vi "主程序-复材超声C扫缺陷分析评定软件.vi"() -> ()   [LabVIEW 2018]
doc: "使用该模板构建用户界面事件处理设计模式。将模板应用于对话框及其它用户界面。用户也可创建并执行VI可按照与用户界面事件相同方式处理的用户定义事件。"
uses:
  <vilib>/Utility/NIReport.llb/Report Type.ctl
  <vilib>/addons/_office/_exclsub.llb/font.ctl
  <vilib>/Utility/NIReport.llb/HTML Report Image Alignment.ctl
  <vilib>/Utility/NIReport.llb/Append Report Text (str wrap).vi
  <vilib>/Utility/NIReport.llb/Append Image to Report (path wrap).vi
  <vilib>/addons/_office/word.llb/Word Easy Table (str).vi
  <vilib>/Utility/NIReport.llb/NI_report.lvclass
  <vilib>/Utility/NIReport.llb/Word/NI_Word.lvclass
  <vilib>/addons/_office/NI_ReportGenerationToolkit.lvlib
  <vilib>/Utility/NIReport.llb/NI_ReportGenerationCore.lvlib
  <vilib>/vision/NI_Vision_Development_Module.lvlib
panel:
  out "flag数组":i8[](array[numeric])
  out "字符串":string
  out "图像Y向分辨率（mm/像素）":dbl
  out "图像X向分辨率（mm/像素）":dbl
  out "判定为筋条的长宽比阈值":i32
  out "框号字体大小-":i16
  out "是否需要预处理":u16
  out "计入缺陷的Z值阈值":i32 caption="值"
  out "计入缺陷的面积阈值":i32
  out "报告模式":string
  in  "删除标注":bool caption="定量分析"
  out "缺陷灰度阈值":dbl caption="值"
  out "穿透图原始路径":path
  out "ROImask":T1(plugin-control)
  out "添加的路径":path
  out "连接的字符串 2":string
  out "临界面积百分比值":dbl
  out "临界Z值":i32
  out "标注后的图片路径":path
  out "全部检测结果合并":string[][](table)
  out "全部检测结果":string[][](table)
  out "部位信息":string[](array[string])=["", "34.500000", "32.500000", "1121", "34", "54.955926", "分层类", "不合格", ""]
  in  "完成标注":bool caption="定量分析"
  out "框数":dbl
  out "自定义字体":T2={"Desired Font (Application)"=enum."Application Font", "[User-specified Font]"={"Font Name"="", "Size"=12, "Strikeout?"=FALSE, "Italic?"=FALSE, "Underline?"=FALSE, "Outline?"=FALSE, "Shadow?"=FALSE, "Bold?"=FALSE, "Rotation Angle"=0.0}, "Horizontal Alignment"=0, "Vertical Alignment"=0} {"Horizontal Alignment" items=["Left", "Center", "Right"]; "Vertical Alignment" items=["Bottom", "Top", "Baseline"]}
  out "框组":T3(array[cluster])
  out "质量等级":string
  in  "stop":bool caption="停止"
  in  "导入图像":bool caption="导入图片"
  in  "开始标注":bool caption="定量分析"
  in  "查看评定结果":bool caption="辅助定性分析"
  in  "生成报告":bool caption="生成原始记录"
  in  "控件":enum32{"穿透图"}(tab)
  out "穿透图":T1(plugin-control)
  out "产品规格":cluster{"产品长度（周长）（mm）":dbl, "产品宽度（母线长）（mm）":dbl}
  out "图像分辨率":T4
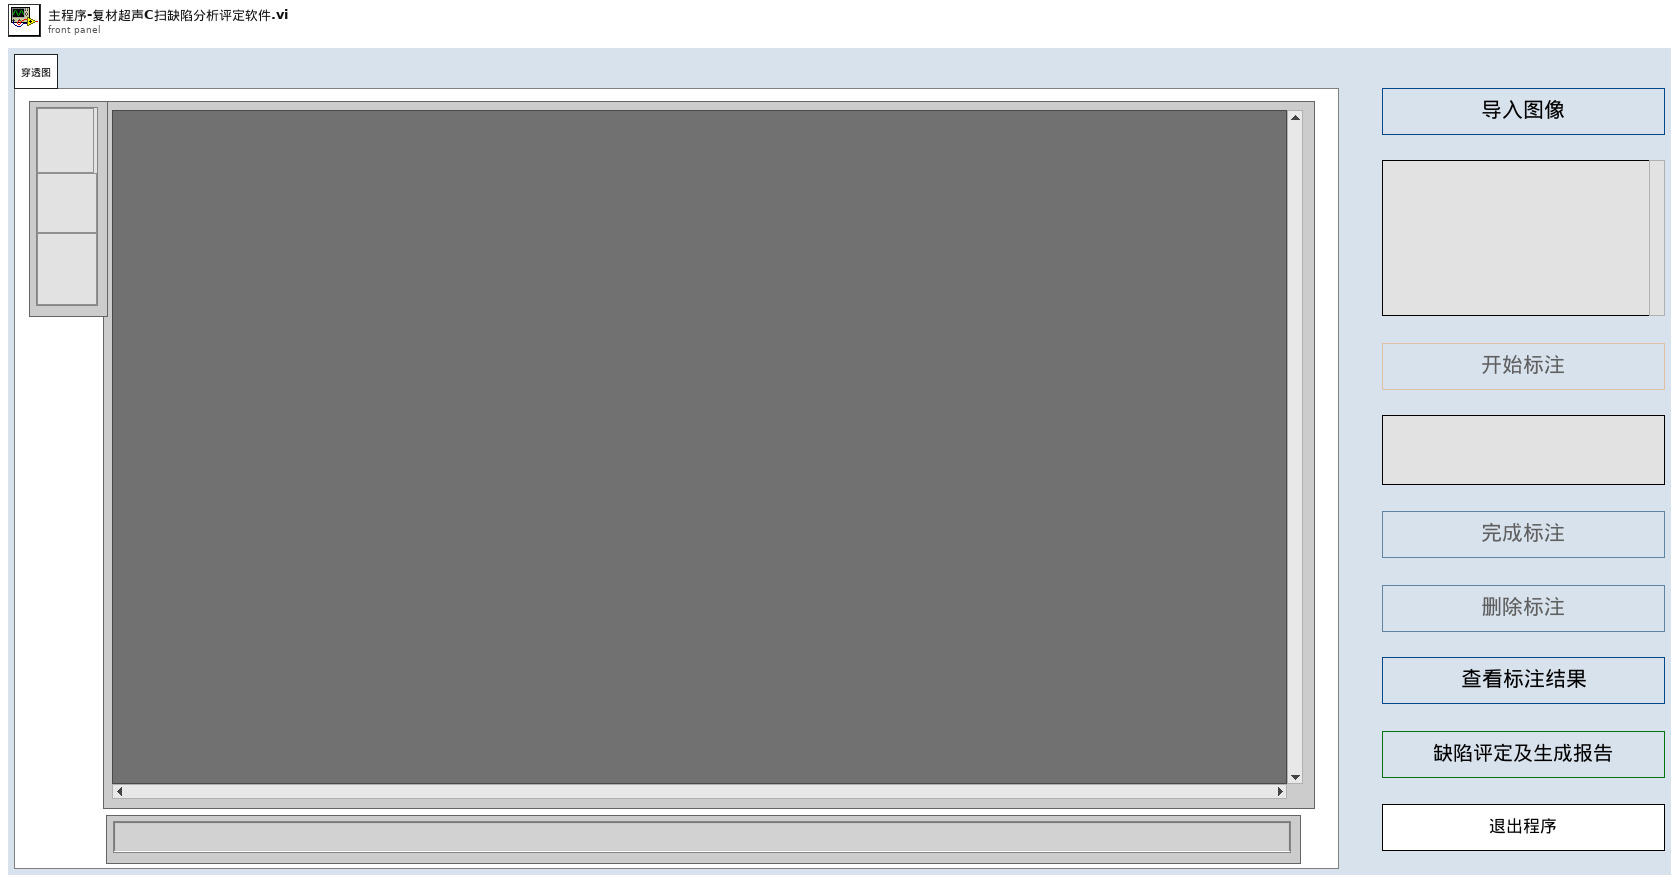
[diagram p1: front panel]
types:
  T1 = typedef "IMAQ Image.ctl" = refnum<image>
  T2 = cluster{"Desired Font (Application)":enum16{"User-specified Font", "Application Font", "System Font", "Dialog Font"}, "[User-specified Font]":cluster{"Font Name":string, "Size":i16, "Strikeout?":bool, "Italic?":bool, "Underline?":bool, "Outline?":bool, "Shadow?":bool, "Bold?":bool, "Rotation Angle":dbl}, "Horizontal Alignment":i16, "Vertical Alignment":i16}
  T3 = cluster{"Global Rectangle":i32[], "Contours":cluster{"Contour Type":u32, "ROI Type":u32, "Points":i32[]}[]}[]
  T4 = cluster{"图像X向分辨率（mm/像素）":dbl, "图像Y向分辨率（mm/像素）":dbl}
  T5 = enum8{"Enabled", "Disabled", "Disabled and Grayed Out"}
  T6 = cluster{"Global Rectangle":i32[], "Contours":cluster{"Contour Type":u32, "ROI Type":u32, "Points":i32[]}[]}
  T7 = cluster{"Zoom Tool":bool, "Selection Tool":bool, "Pan Tool":bool, "Point Tool":bool, "Line Tool":bool, "Rectangle Tool":bool, "Rotated Rectangle Tool":bool, "Polyline Tool":bool, "Polygon Tool":bool, "Freehand Tool":bool, "Closed Freehand Tool":bool, "Ellipse Tool":bool, "Annulus Tool":bool}
  T8 = enum16{"maximized", "minimized", "normal", "no change"}
  T9 = typedef "NI_ReportGenerationCore.lvlib/Report Type.ctl" = enum16{"HTML", "Word", "Excel"}
  T10 = typedef "NI_ReportGenerationCore.lvlib/HTML Report Image Alignment.ctl" = enum16{"(default)", "LEFT", "RIGHT", "TOP", "TEXTTOP", "MIDDLE", "ABSMIDDLE", "BASELINE", "BOTTOM", "ABSBOTTOM"}
  T11 = cluster{"position (Excel)":cluster{"row":i32, "column":i32}, "name (Excel)":string, "bookmark (Word)":string}
  T12 = cluster{"position (excel)":cluster{"row":i32, "column":i32}, "name (excel)":string, "bookmark (word)":string}
  T13 = typedef "NI_ReportGenerationToolkit.lvlib/font.ctl" = cluster{"font name":string, "font size":dbl, "bold":u16, "italic":u16, "underline":u16, "strike through":u16, "font color":u32}
  T14 = typedef "Image Type" = u32
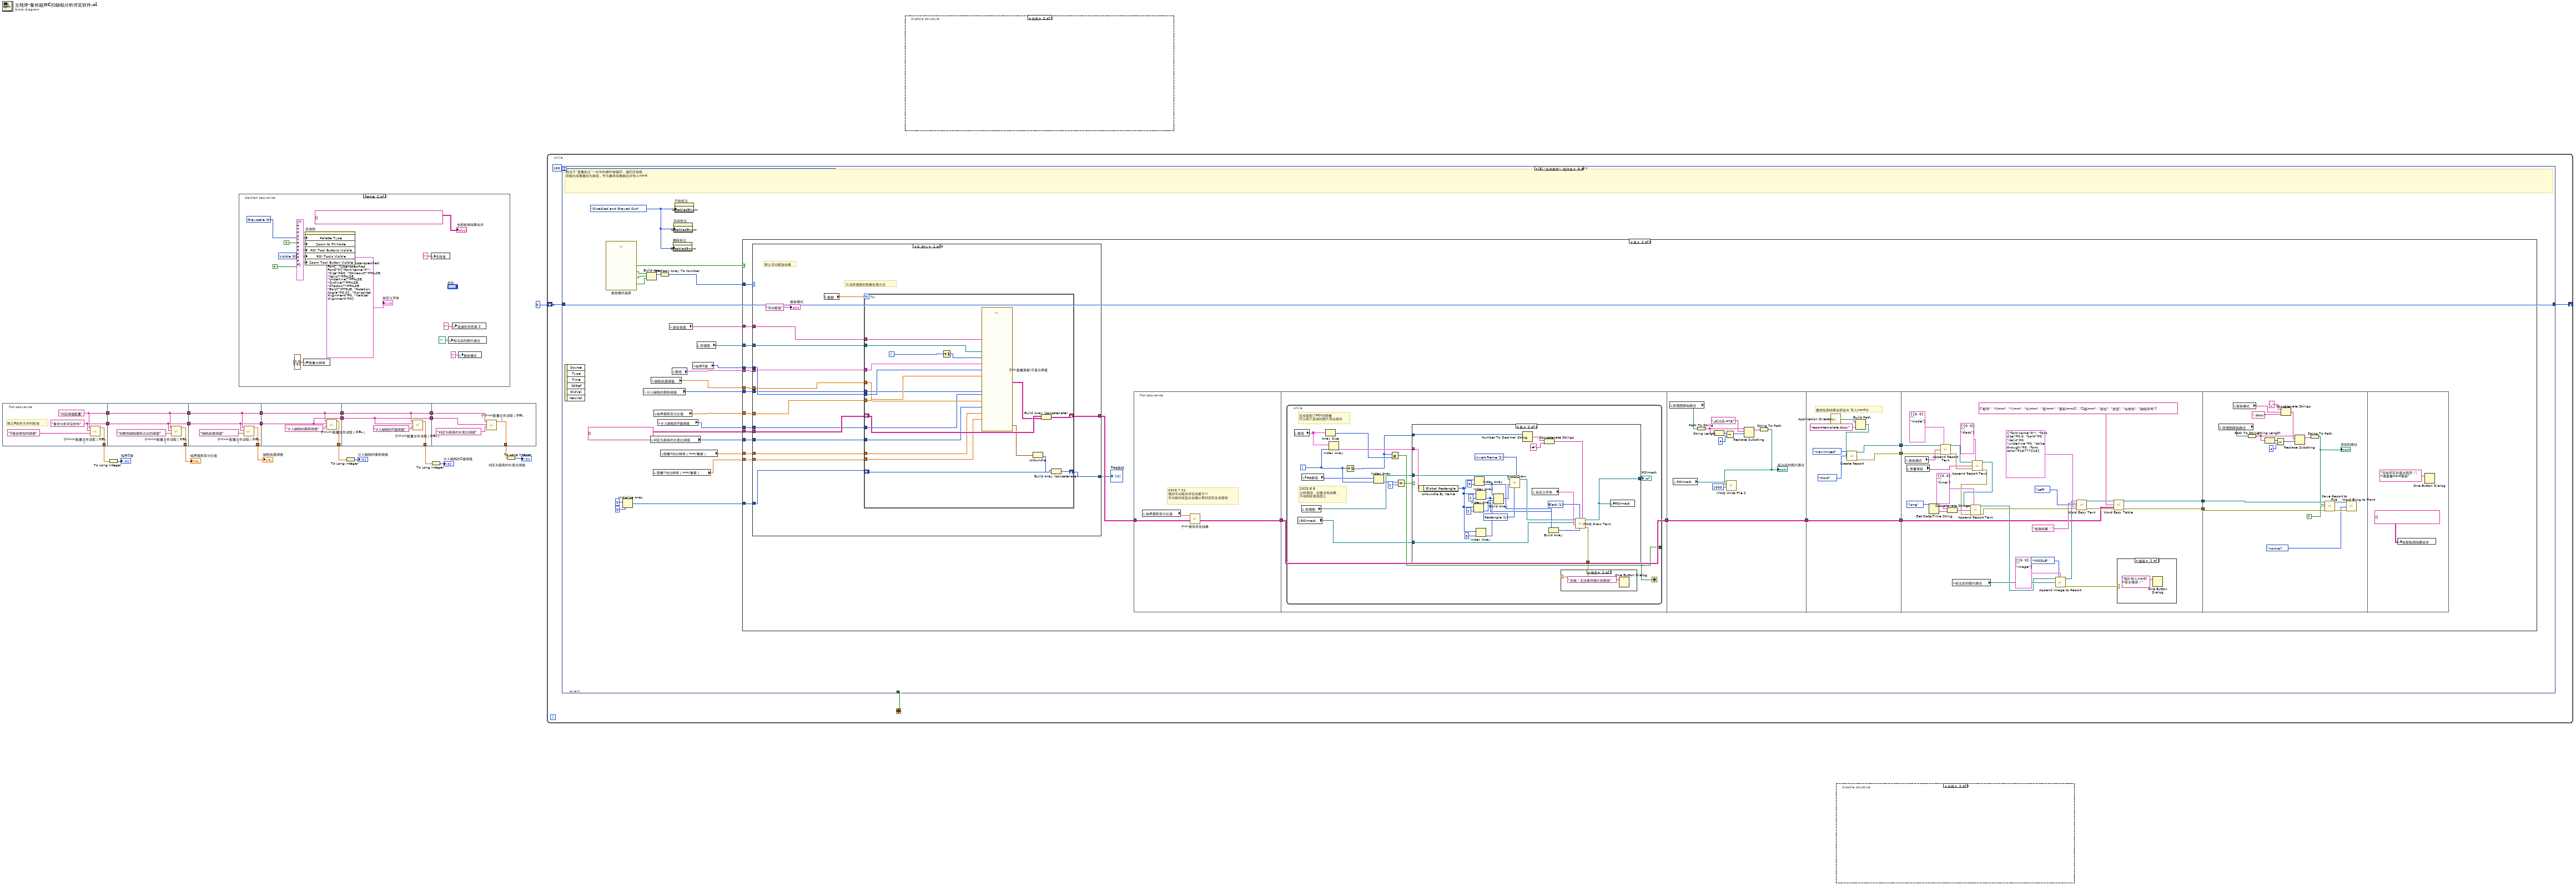
[diagram p0: block diagram]
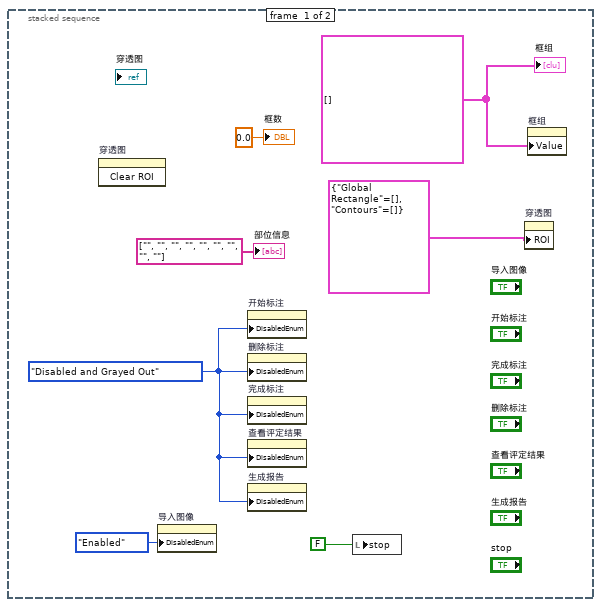
[diagram p3: hidden frame]
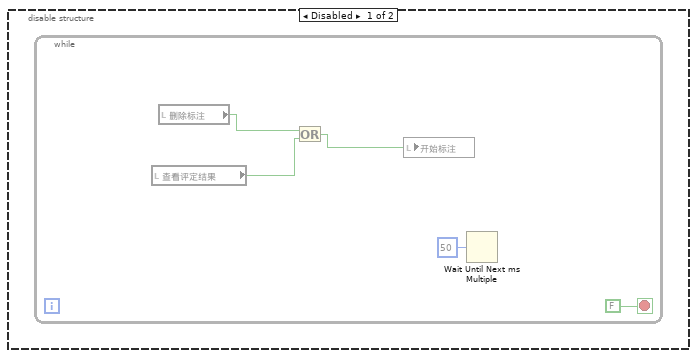
[diagram p4: hidden frame]
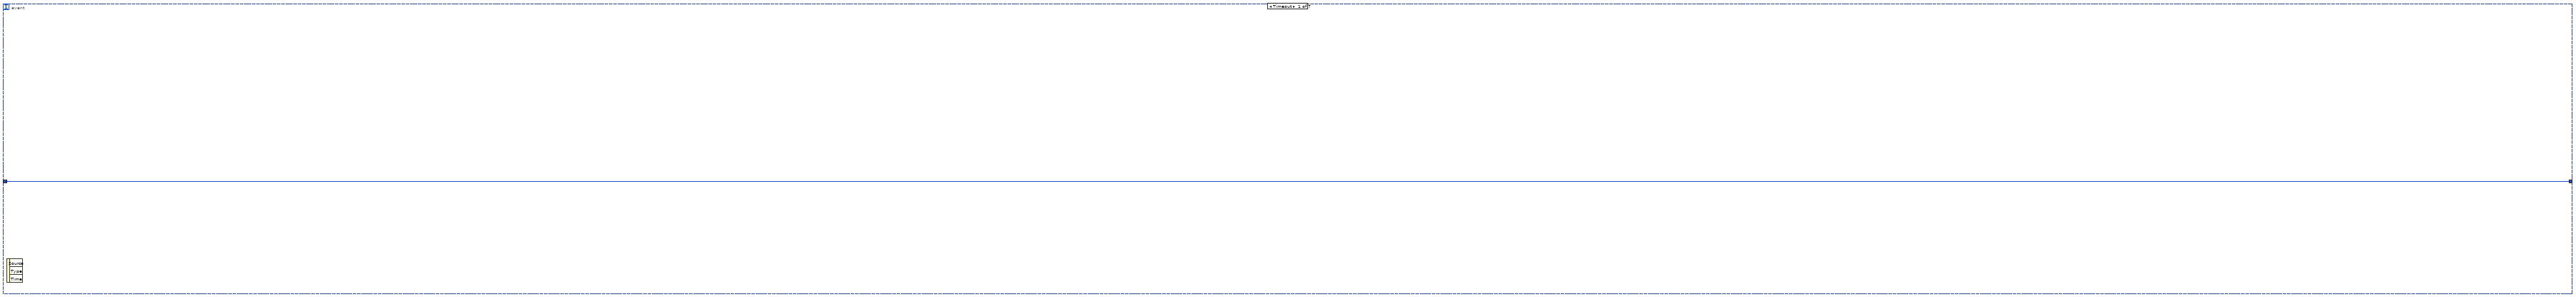
[diagram p5: hidden frame]
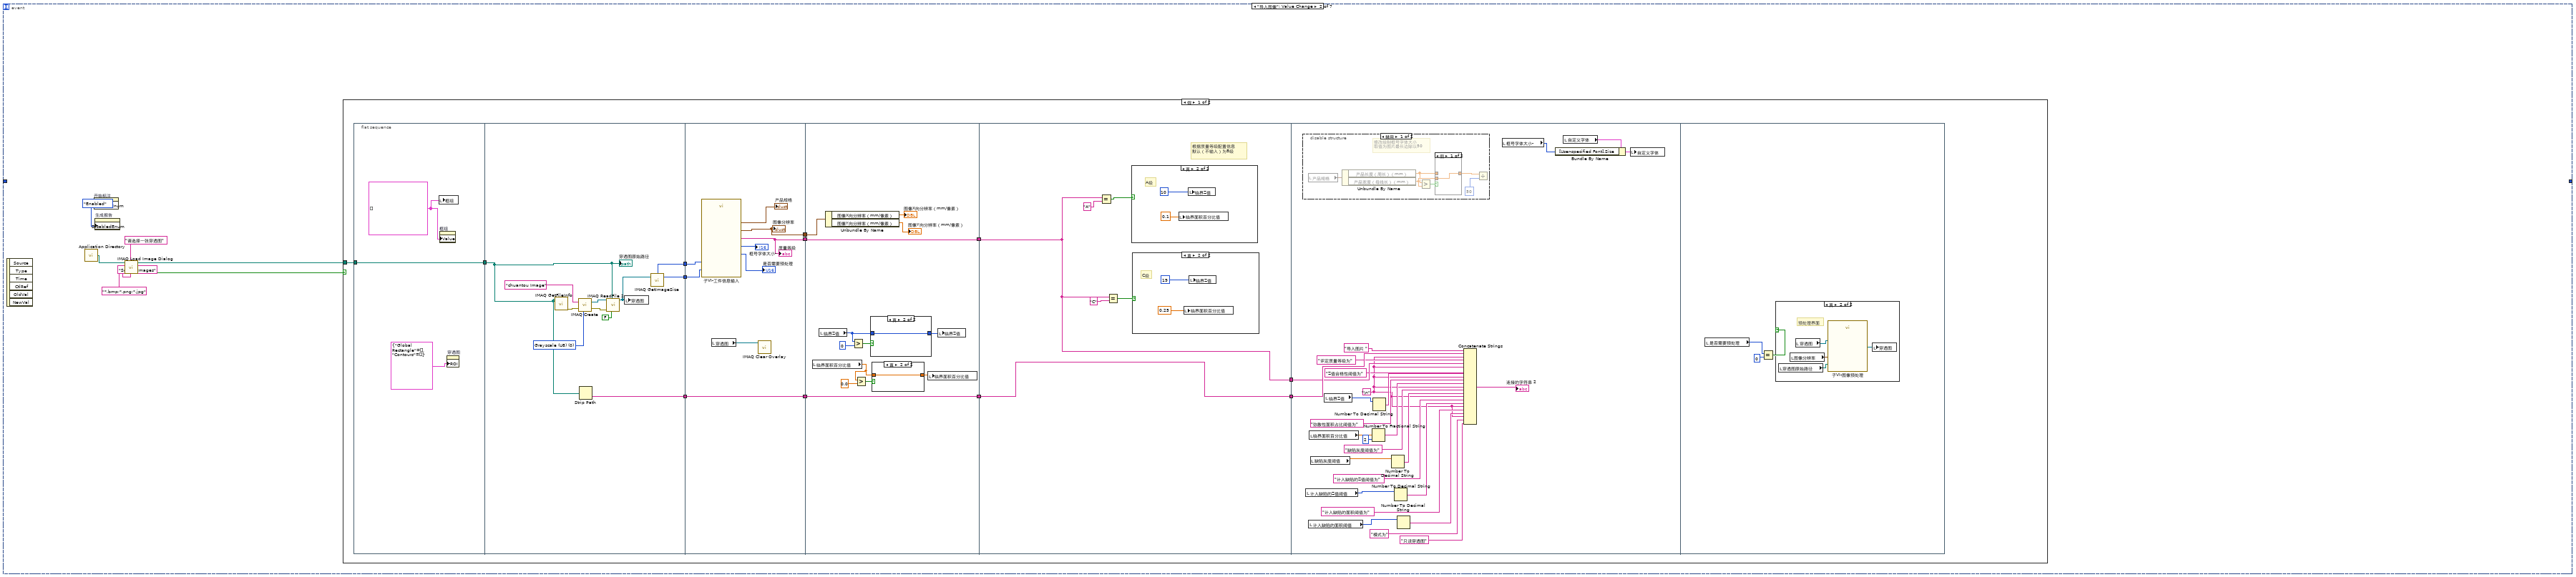
[diagram p6: hidden frame]
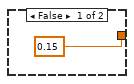
[diagram p7: hidden frame]
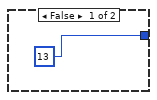
[diagram p8: hidden frame]
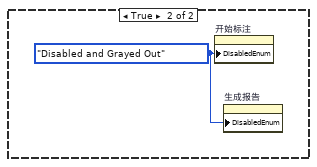
[diagram p14: hidden frame]
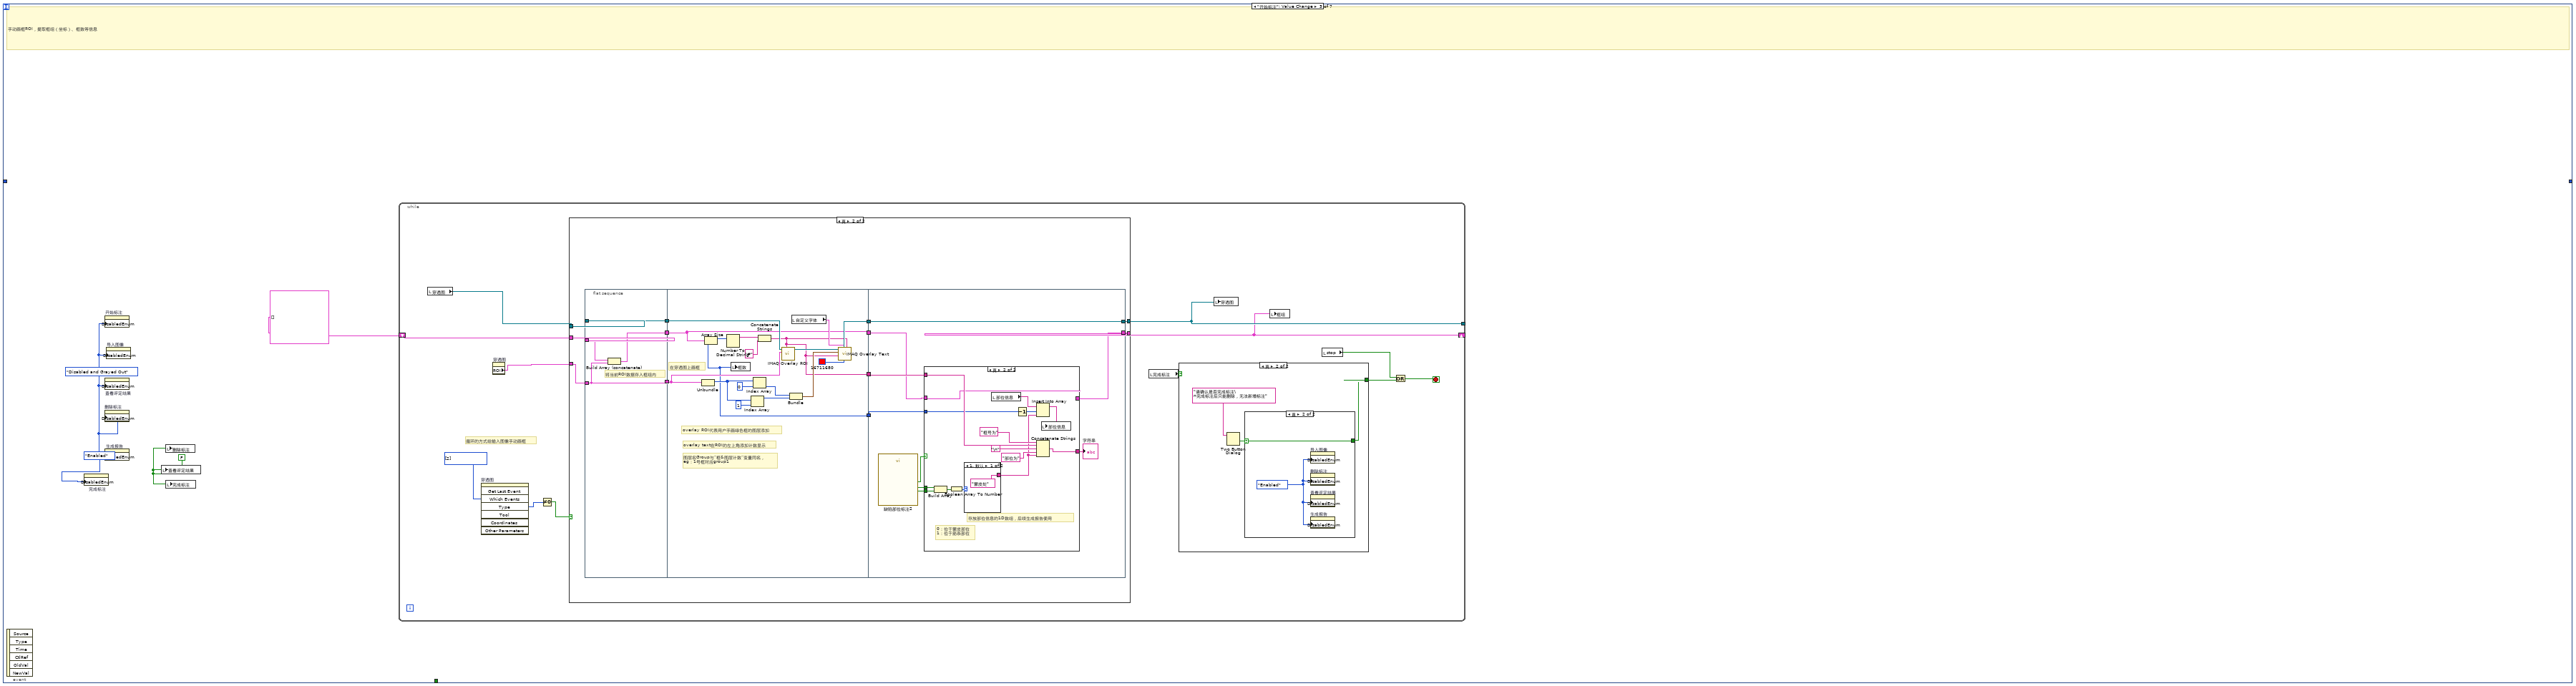
[diagram p15: hidden frame]
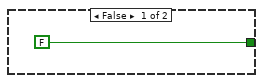
[diagram p16: hidden frame]
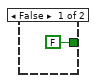
[diagram p17: hidden frame]
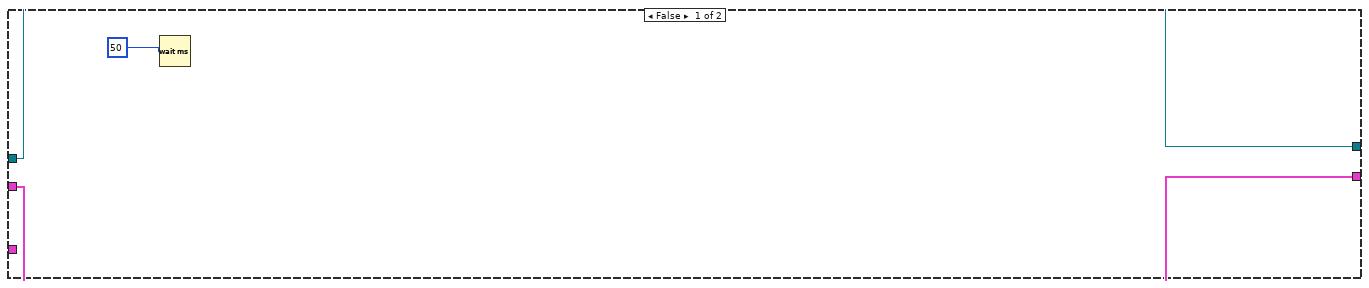
[diagram p18: hidden frame]
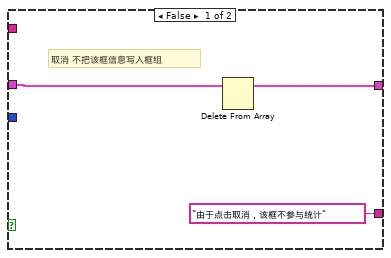
[diagram p19: hidden frame]
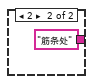
[diagram p20: hidden frame]
diagram:
  n1 = flat-sequence {
    tunnel: [w24] -> w20
    tunnel: [w23] -> w19
    tunnel: [w22] -> w14
    tunnel: w20 -> [w27]
    tunnel: w19 -> [w28]
    tunnel: [w28] -> w18
    tunnel: [w27] -> w17
    tunnel: [w26] -> w15
    tunnel: w18 -> [w30]
    tunnel: w17 -> [w31]
    tunnel: [w32] -> w16
    tunnel: [w31] -> w12
    tunnel: [w30] -> w11
    tunnel: w12 -> [w35]
    tunnel: w11 -> [w34]
    tunnel: [w36] -> w9
    tunnel: [w35] -> w8
    tunnel: [w34] -> w7
    tunnel: w8 -> [w39]
    tunnel: w7 -> [w38]
    tunnel: [w40] -> w5
    tunnel: [w39] -> w4
    tunnel: [w38] -> w3
    tunnel: w4 -> [w45]
    tunnel: w3 -> [w44]
    tunnel: [w42] -> w2
    frame #0 {
      w23 = "复材分析评定软件" ("section")
      w24 = "判定阈值配置" ("文件名称")
      # "默认B级作为评判标准"
      n2 = call "子VI-ini配置文件读取（DBL）.vi"("key"="Z值合格性的阈值", "section"=w23, "文件名称"=w24) -> ("value"=w22:dbl)  [unwired: 8 in]
    }
    frame #1 {
      n3 = call "子VI-ini配置文件读取（DBL）.vi"("key"="弥散性缺陷面积占比的阈值", "section"=w28, "文件名称"=w27) -> ("value"=w26:dbl)  [unwired: 8 in]
    }
    frame #2 {
      n4 = call "子VI-ini配置文件读取（DBL）.vi"("key"="缺陷灰度阈值", "section"=w30, "文件名称"=w31) -> ("value"=w32:dbl)  [unwired: 8 in]
    }
    frame #3 {
      n5 = call "子VI-ini配置文件读取（DBL）.vi"("key"="计入缺陷的面积阈值", "section"=w34, "文件名称"=w35) -> ("value"=w36:dbl)  [unwired: 8 in]
    }
    frame #4 {
      n6 = call "子VI-ini配置文件读取（DBL）.vi"("key"="计入缺陷的Z值阈值", "section"=w38, "文件名称"=w39) -> ("value"=w40:dbl)  [unwired: 8 in]
    }
    frame #5 {
      n7 = call "子VI-ini配置文件读取（DBL）.vi"("key"="判定为筋条的长宽比阈值", "section"=w44, "文件名称"=w45) -> ("value"=w42:dbl)  [unwired: 8 in]
    }
  }
  n8 = To Long Integer(number=w14) -> (32bit integer=→"临界Z值":i32)
  n9 = stacked-sequence {
    frame #0 {
      w50 = T3 [] ("框组")
      w48 = T5."Disabled and Grayed Out" ("禁用")
      n10 = invoke on="穿透图" class="ImageControl" method="Clear ROI"() -> ()  [unwired: 3 in, 3 out]
      n11 = property on="导入图像" class="Bool"("DisabledEnum"=T5."Enabled" ("禁用")) -> ()  [unwired: 2 in, 2 out]
      n12 = property on="开始标注" class="Bool"("DisabledEnum"=w48) -> ()  [unwired: 2 in, 2 out]
      n13 = property on="删除标注" class="Bool (严格)"("DisabledEnum"=w48) -> ()  [unwired: 2 in, 2 out]
      n14 = property on="完成标注" class="Bool (严格)"("DisabledEnum"=w48) -> ()  [unwired: 2 in, 2 out]
      n15 = property on="查看评定结果" class="Bool (严格)"("DisabledEnum"=w48) -> ()  [unwired: 2 in, 2 out]
      n16 = property on="生成报告" class="Bool"("DisabledEnum"=w48) -> ()  [unwired: 2 in, 2 out]
      n17 = local write "stop"(FALSE ("stop")) -> ()
      n18 = property on="穿透图" class="ImageControl"("ROI"=T6 {"Global Rectangle"=[], "Contours"=[]}) -> ()  [unwired: 2 in, 2 out]
      n19 = property on="框组" class="Arr (严格)"("Value"=w50) -> ()  [unwired: 2 in, 2 out]
      "部位信息" <- string[] ["", "", "", "", "", "", "", "", ""] ("部位信息")
      "框组" <- w50
      "框数" <- 0.0 ("框数")
    }
    frame #1 {
      w54 = u32 0 items=["Visible", "Hidden", "Hidden, Use WindTools Palette"] ("ROI Tools Visible")
      w57 = u32 0 items=["Grayscale", "Binary", "Gradient", "Rainbow", "Temperature", "User Defined", "Binary 16 Bit", "Gradient 16 Bit", "Rainbow 16 Bit", "Temperature 16 Bit", "User Defined 16 Bit"] ("Palette:Palette Type")
      n20 = local write "图像分辨率"(T4 {"图像X向分辨率（mm/像素）"=1.0, "图像Y向分辨率（mm/像素）"=1.0} ("图像分辨率")) -> ()
      n21 = property on="穿透图" class="ImageControl"("Palette Type"=w57, "Zoom to Fit Mode"=TRUE, "ROI Tool Buttons Visible"=T7 {"Zoom Tool"=TRUE, "Selection Tool"=FALSE, "Pan Tool"=TRUE, "Point Tool"=FALSE, "Line Tool"=FALSE, "Rectangle Tool"=TRUE, "Rotated Rectangle Tool"=FALSE, "Polyline Tool"=FALSE, "Polygon Tool"=FALSE, "Freehand Tool"=FALSE, "Closed Freehand Tool"=FALSE, "Ellipse Tool"=FALSE, "Annulus Tool"=FALSE} ("ROI Tool Buttons Visible:All Elements"), "ROI Tools Visible"=w54, "Zoom Tool Button Visible"=TRUE ("ROI Tool Buttons Visible:Zoom Tool Button Visible")) -> ()  [unwired: 2 in, 2 out]
      n22 = local write "字符串"("" ("字符串")) -> ()
      n23 = local write "标注后的图片路径"(path "" ("标注后的图片路径")) -> ()
      n24 = local write "连接的字符串 2"("" ("连接的字符串 2")) -> ()
      n25 = local write "报告模式"("" ("报告模式")) -> ()
      "自定义字体" <- T2 {"Desired Font (Application)"=enum."User-specified Font", "[User-specified Font]"={"Font Name"="", "Size"=60, "Strikeout?"=FALSE, "Italic?"=FALSE, "Underline?"=FALSE, "Outline?"=FALSE, "Shadow?"=FALSE, "Bold?"=TRUE, "Rotation Angle"=0.0}, "Horizontal Alignment"=0, "Vertical Alignment"=0} ("Font, Size & Style")
      "全部检测结果合并" <- string[][] [] ("弥散类检测结果合并")
    }
  }
  n26 = To Long Integer(number=w9) -> (32bit integer=→"计入缺陷的面积阈值":i32)
  n27 = To Long Integer(number=w5) -> (32bit integer=→"计入缺陷的Z值阈值":i32)
  n28 = To Long Integer(number=w2) -> (32bit integer=→"判定为筋条的长宽比阈值":i32)
  n29 = while {
    shift-right: [w65] -> _
    shift-left: 0 -> [w66]
    stop <- w68 stop-if-true
    n30 = event shown="[5] \"生成报告\": 值改变" {
      selector: _ -> [_ _ _ _ _ _ _]
      dyn-events: _ -> [_ _ _ _ _ _ _]
      timeout: 100 -> [_ _ _ _ _ _ _]
      tunnel: [_ _ _ _ _ _ w585] -> w68
      tunnel: w66 -> [w69 _ _ _ _ w339 _]
      tunnel: [w69 _ _ _ _ w339 0] -> w65
      event Timeout {
        n31 = event-data() -> ()  [unwired: 1 in, 3 out]
      }
      event "导入图像": Value Change {
        w71 = T5."Enabled" ("禁用")
        n32 = event-data() -> ()  [unwired: 1 in, 6 out]
        n33 = call <vilib>:"Application Directory.vi"() -> ("Application Directory"=w70:path)
        n34 = property on="开始标注" class="Bool"("DisabledEnum"=w71) -> ()  [unwired: 2 in, 2 out]
        n35 = property on="生成报告" class="Bool"("DisabledEnum"=w71) -> ()  [unwired: 2 in, 2 out]
        n36 = call "IMAQ Load Image Dialog"("Pattern Label"="Source Images", "Prompt"="请选择一张穿透图" ("prompt"), "Pattern"="*.bmp;*.png;*.jpg", "Start Path"=w70) -> ("Cancelled?"=w73:bool, "Path"=w72:path)  [unwired: 5 in, 1 out]
        n37 = case shown="假" w73 {
          tunnel: w72 -> [w86 _]
          frame False {
            n38 = flat-sequence {
              tunnel: w86 -> [w90]
              tunnel: [w90] -> w85
              tunnel: w85 -> [w93]
              tunnel: [w95] -> w84
              tunnel: [w94] -> w83
              tunnel: [w92] -> w82
              tunnel: [w110] -> w88
              tunnel: w84 -> [w109]
              tunnel: w83 -> [w108]
              tunnel: w82 -> [w107]
              tunnel: [w107] -> w81
              tunnel: [w103] -> w77
              tunnel: w88 -> [w124]
              tunnel: [w124] -> w87
              tunnel: w81 -> [w123]
              tunnel: [w123] -> w80
              tunnel: w77 -> [w114]
              tunnel: w87 -> [w129]
              tunnel: w80 -> [w130]
              tunnel: [w130] -> w79
              tunnel: [w129] -> w78
              tunnel: w79 -> [w156]
              tunnel: w78 -> [w154]
              frame #0 {
                w91 = T3 [] ("框组")
                n39 = local write "框组"(w91) -> ()
                n40 = property on="框组" class="Arr (严格)"("Value"=w91) -> ()  [unwired: 2 in, 2 out]
                n41 = property on="穿透图" class="ImageControl"("ROI"=T6 {"Global Rectangle"=[], "Contours"=[]}) -> ()  [unwired: 2 in, 2 out]
              }
              frame #1 {
                w97 = T14 0 items=["Grayscale (U8)", "Grayscale (I16)", "Grayscale (SGL)", "Complex (CSG)", "RGB (U32)", "HSL (U32)", "RGB (U64)", "Grayscale (U16)"] ("Image Type")
                n42 = call "IMAQ GetFileInfo"("File Path"=w93) -> ("error out"=w100:errorcluster)  [unwired: 4 in, 6 out]
                n43 = call "IMAQ Create"("Image Name"="chuantou Image", "Image Type"=w97, "error in (no error)"=w100) -> ("New Image"=w101:T1, "error out"=w102:errorcluster)  [unwired: 2 in]
                n44 = Strip Path(path=w93) -> (name=w92:string)  [unwired: 1 out]
                n45 = call "IMAQ ReadFile 2"("Use File Path Image Type"=FALSE, "File Path"=w93, "error in (no error)"=w102, "Image"=w101) -> ("Image Out"=w99:T1)  [unwired: 3 in, 4 out]
                n46 = local write "穿透图"(w99) -> ()
                n47 = call "IMAQ GetImageSize"("Image"=w99) -> ("Y Resolution"=w94:i32, "X Resolution"=w95:i32)  [unwired: 3 in, 1 out]
                "穿透图原始路径" <- w93
              }
              frame #2 {
                n48 = call "子VI-工件信息输入.vi"("Y Resolution"=w108, "X Resolution"=w109) -> ("质量等级"=w110:string, "框号字体大小-"=→"框号字体大小-":i16, "产品规格"=→"产品规格":cluster{"产品长度（周长）（mm）":dbl, "产品宽度（母线长）（mm）":dbl}, "是否需要预处理"=→"是否需要预处理":u16, "图像分辨率"=w103:T4)  [unwired: 5 in]
                "图像分辨率" <- w103
                "质量等级" <- w110
                n49 = local read "穿透图"() -> (w106:T1)
                n50 = call "IMAQ Clear Overlay"("Image"=w106) -> ()  [unwired: 9 in, 2 out]
              }
              frame #3 {
                n51 = local read "临界面积百分比值"() -> (w115:dbl)
                n52 = local read "临界Z值"() -> (w116:i32)
                n53 = Unbundle By Name(w114) -> ("图像X向分辨率（mm/像素）"=→"图像X向分辨率（mm/像素）":dbl, "图像Y向分辨率（mm/像素）"=→"图像Y向分辨率（mm/像素）":dbl)
                n54 = Greater?(x=w116, y=0) -> (0:w121:bool)
                n55 = Greater?(x=w115, y=0.0) -> (0:w119:bool)
                n56 = case shown="真" w121 {
                  tunnel: [13 ("临界Z值") w128] -> w118
                  tunnel: w116 -> [_ w128]
                  frame False {
                  }
                  frame True {
                  }
                }
                n57 = case shown="真" w119 {
                  tunnel: [0.15 ("临界面积百分比值") w126] -> w117
                  tunnel: w115 -> [_ w126]
                  frame False {
                  }
                  frame True {
                  }
                }
                n58 = local write "临界面积百分比值"(w117) -> ()
                n59 = local write "临界Z值"(w118) -> ()
              }
              frame #4 {
                # "根据质量等级配置信息\n默认（不输入）为B级"
                n60 = Equal?(x=w129, y="A") -> (x = y?=w133:bool)
                n61 = Equal?(x=w129, y="C") -> (x = y?=w134:bool)
                n62 = case shown="真" w133 {
                  frame False {
                  }
                  frame True {
                    # "A级"
                    n63 = local write "临界面积百分比值"(0.1 ("临界面积百分比值")) -> ()
                    n64 = local write "临界Z值"(10 ("临界Z值")) -> ()
                  }
                }
                n65 = case shown="真" w134 {
                  frame False {
                  }
                  frame True {
                    # "C级"
                    n66 = local write "临界面积百分比值"(0.25 ("临界面积百分比值")) -> ()
                    n67 = local write "临界Z值"(19 ("临界Z值")) -> ()
                  }
                }
              }
              frame #5 {
                w144 = "\n"
                n68 = disable-structure shown="禁用" {
                  frame Disabled {
                    # "修改绘制框号字体大小\n取值为图片最长边除以50"
                    n69 = local read "产品规格"() -> (w167:cluster{"产品长度（周长）（mm）":dbl, "产品宽度（母线长）（mm）":dbl})
                    n70 = Unbundle By Name(w167) -> ("产品长度（周长）（mm）"=w169:dbl, "产品宽度（母线长）（mm）"=w170:dbl)
                    n71 = Greater?(x=w169, y=w170) -> (0:w168:bool)
                    n72 = case shown="假" w168 {
                      tunnel: w169 -> [_ w173]
                      tunnel: w170 -> [w172 _]
                      tunnel: [w172 w173] -> w171
                      frame False {
                      }
                      frame True {
                      }
                    }
                    n73 = Divide(x=w171, y=i8 50) -> ()  [unwired: 1 out]
                  }
                  frame Enabled {
                  }
                }
                n74 = local read "计入缺陷的Z值阈值"() -> (w150:i32)
                n75 = local read "计入缺陷的面积阈值"() -> (w147:i32)
                n76 = local read "临界面积百分比值"() -> (w162:dbl)
                n77 = local read "缺陷灰度阈值"() -> (w164:dbl)
                n78 = local read "临界Z值"() -> (w160:i32)
                n79 = Number To Fractional String(number=w162, precision (6)=i16 2 ("精度(6)")) -> (F-format string=w163:string)  [unwired: 2 in]
                n80 = Number To Decimal String(number=w160) -> (decimal integer string=w161:string)  [unwired: 1 in]
                n81 = Number To Decimal String(number=w164) -> (decimal integer string=w165:string)  [unwired: 1 in]
                n82 = Number To Decimal String(number=w150) -> (decimal integer string=w148:string)  [unwired: 1 in]
                n83 = Number To Decimal String(number=w147) -> (decimal integer string=w145:string)  [unwired: 1 in]
                n84 = Concatenate Strings("导入图片 " ("字符串"), w156, w144, "评定质量等级为" ("字符串"), w154, w144, "Z值合格性阈值为" ("字符串"), w161, w144, "弥散性面积占比阈值为" ("字符串"), w163, w144, "缺陷灰度阈值为" ("字符串"), w165, w144, "计入缺陷的Z值阈值为" ("字符串"), w148, w144, "计入缺陷的面积阈值为" ("字符串"), w145, w144, "模式为" ("字符串"), "只读穿透图" ("字符串")) -> (→"连接的字符串 2":string)
                n85 = local read "框号字体大小-"() -> (w140:i16)
                n86 = local read "自定义字体"() -> (w141:T2)
                n87 = Bundle By Name(cluster=w141, "[User-specified Font].Size"=w140) -> (w142:T2)
                n88 = local write "自定义字体"(w142) -> ()
              }
              frame #6 {
                n89 = local read "是否需要预处理"() -> (w175:u16)
                n90 = Equal?(x=w175, y=u16 0) -> (x = y?=w176:bool)
                n91 = case shown="真" w176 {
                  frame False {
                  }
                  frame True {
                    # "预处理界面"
                    n92 = local read "穿透图原始路径"() -> (w177:path)
                    n93 = local read "图像分辨率"() -> (w178:T4)
                    n94 = local read "穿透图"() -> (w180:T1)
                    n95 = call "子VI-图像预处理.vi"("图像分辨率"=w178, "穿透图"=w180, "穿透图原始路径"=w177) -> ("穿透图out"=w179:T1)  [unwired: 8 in]
                    n96 = local write "穿透图"(w179) -> ()
                  }
                }
              }
            }
          }
          frame True {
            w181 = T5."Disabled and Grayed Out" ("禁用")
            n97 = property on="开始标注" class="Bool"("DisabledEnum"=w181) -> ()  [unwired: 2 in, 2 out]
            n98 = property on="生成报告" class="Bool"("DisabledEnum"=w181) -> ()  [unwired: 2 in, 2 out]
          }
        }
      }
      event "开始标注": Value Change {
        w183 = T5."Disabled and Grayed Out" ("禁用")
        w185 = FALSE ("完成标注")
        # "手动画框ROI，提取框组（坐标）、框数等信息"
        n99 = event-data() -> ()  [unwired: 1 in, 6 out]
        n100 = property on="完成标注" class="Bool (严格)"("DisabledEnum"=T5."Enabled" ("禁用")) -> ()  [unwired: 2 in, 2 out]
        n101 = property on="查看评定结果" class="Bool (严格)"("DisabledEnum"=w183) -> ()  [unwired: 2 in, 2 out]
        n102 = property on="删除标注" class="Bool (严格)"("DisabledEnum"=w183) -> ()  [unwired: 2 in, 2 out]
        n103 = property on="生成报告" class="Bool"("DisabledEnum"=w183) -> ()  [unwired: 2 in, 2 out]
        n104 = property on="开始标注" class="Bool"("DisabledEnum"=w183) -> ()  [unwired: 2 in, 2 out]
        n105 = property on="导入图像" class="Bool"("DisabledEnum"=w183) -> ()  [unwired: 2 in, 2 out]
        n106 = local write "查看评定结果"(w185) -> ()
        n107 = local write "删除标注"(w185) -> ()
        n108 = local write "完成标注"(w185) -> ()
        n109 = while {
          shift-right: [w190] -> _
          shift-left: T3 [] ("框组") -> [w197]
          tunnel: [w195] -> _
          stop <- w189 stop-if-true
          (unwired) "_" ("名称或相对路径")
          (unwired) ".docx" ("名称或相对路径")
          w188 = i32[] [2] items=["No Event"=0, "Click Event"=1, "Draw Event"=2, "Size Event"=4, "Scroll Event"=5, "Double Click Event"=8] ("Which Events")
          # "循环的方式给输入图像手动画框"
          n110 = local read "穿透图"() -> (w196:T1)
          n111 = invoke on="穿透图" class="ImageControl" method="Get Last Event"("Which Events"=w188) -> ("Type"=w187:i32)  [unwired: 7 in, 7 out]
          n112 = property on="穿透图" class="ImageControl"() -> ("ROI"=w186:T6)  [unwired: 2 in, 2 out]
          n113 = Not Equal To 0?(x=w187) -> (x != 0?=w191:bool)
          n114 = case shown="真" w191 {
            tunnel: w196 -> [w208 w220]
            tunnel: [w208 w219] -> w195
            tunnel: [w206 w217] -> w190
            tunnel: w197 -> [w206 w218]
            tunnel: w186 -> [_ w216]
            frame False {
              n115 = Wait (ms)(milliseconds to wait=u32 50 ("毫秒倍数")) -> ()  [unwired: 1 out]
              n116 = Wait (ms)(milliseconds to wait=u32 50) -> ()  [unwired: 1 out]
            }
            frame True {
              n117 = flat-sequence {
                tunnel: w220 -> [w221]
                tunnel: [w221] -> w215
                tunnel: w216 -> [w224]
                tunnel: [w224] -> w214
                tunnel: w218 -> [w223]
                tunnel: [w222] -> w213
                tunnel: w215 -> [w233]
                tunnel: w214 -> [w232]
                tunnel: w213 -> [w225]
                tunnel: [w235] -> w212
                tunnel: [w225] -> w211
                tunnel: [w229] -> w210
                tunnel: [w227] -> w209
                tunnel: w212 -> [w250]
                tunnel: w211 -> [w244]
                tunnel: w210 -> [w247]
                tunnel: w209 -> [w246]
                tunnel: [w250] -> w219
                tunnel: [w243] -> w217
                frame #0 {
                  # "将当前ROI数据存入框组内"
                  n118 = Build Array (concatenate)(w223, w224) -> (w222:T3)
                }
                frame #1 {
                  # "在穿透图上画框"
                  # "图层名Group与“框&图层计数”变量同名，\neg：1号框对应group1"
                  # "overlay text在ROI的左上角添加计数显示"
                  # "overlay ROI代表用户手画绿色框的图层添加"
                  n119 = Unbundle(w232) -> ("Global Rectangle"=w240:i32[])  [unwired: 1 out]
                  n120 = Array Size(array=w225) -> (size(s)=w227:i32)
                  n121 = Number To Decimal String(number=w227) -> (decimal integer string=w228:string)  [unwired: 1 in]
                  n122 = local write "框数"(w227) -> ()
                  n123 = Index Array(array=w240, index=1 ("索引")) -> (element=w238:i32)
                  n124 = Index Array(array=w240, index=0 ("索引")) -> (element=w239:i32)
                  n125 = Concatenate Strings(w228, "#" ("字符串")) -> (w229:string)
                  n126 = call "IMAQ Overlay ROI"("Group"=w229, "ROI Descriptor"=w232, "Image"=w233) -> ("Image Out"=w241:T1)  [unwired: 7 in, 1 out]
                  n127 = Bundle(w239, w238) -> (w234:cluster{i32, i32})  [unwired: 1 in]
                  n128 = local read "自定义字体"() -> (w231:T2)
                  n129 = call "IMAQ Overlay Text"("Group"=w229, "Text Color (black)"=u32 16711680, "Font, Size & Style"=w231, "String"=w229, "Origin"=w234, "Image"=w241) -> ("Image Out"=w235:T1)  [unwired: 4 in, 1 out]
                }
                frame #2 {
                  n130 = call "缺陷部位标注2"() -> ("位于筋条处"=w249:bool, "位于蒙皮处"=w248:bool, "确定"=w245:bool)  [unwired: 16 in, 1 out]
                  n131 = case shown="真" w245 {
                    tunnel: w249 -> [_ w266]
                    tunnel: w248 -> [_ w265]
                    tunnel: w247 -> [_ w261]
                    tunnel: w246 -> [_ w258]
                    tunnel: w244 -> [w253 w255]
                    tunnel: [w252 w255] -> w243
                    tunnel: ["由于点击取消，该框不参与统计" w254] -> w242
                    frame False {
                      # "取消 不把该框信息写入框组"
                      n132 = Delete From Array(array=w253) -> (array with subset deleted=w252:T3)  [unwired: 2 in, 1 out]
                    }
                    frame True {
                      # "0：位于蒙皮部位\n1：位于筋条部位"
                      # "存放部位信息的1D数组，后续生成报告使用"
                      n133 = Build Array(w265, w266) -> (w267:bool[])
                      n134 = Boolean Array To Number(Boolean array=w267) -> (number=w268:u32)
                      n135 = case shown="1, 默认" w268 {
                        tunnel: ["蒙皮处" ("t") "筋条处" ("t")] -> w256
                        frame 1, Default {
                        }
                        frame 2 {
                        }
                      }
                      n136 = local read "部位信息"() -> (w260:string[])
                      n137 = Decrement(x=w258) -> (x-1=w257:i32)
                      n138 = Insert Into Array(array=w260, index=w257, new element=w256) -> (w259:string[])
                      n139 = Concatenate Strings("框号为" ("字符串"), w261, "\n", "部位为" ("字符串"), w256) -> (w254:string)
                      n140 = local write "部位信息"(w259) -> ()
                    }
                  }
                  "字符串" <- w242
                }
              }
            }
          }
          n141 = local read "完成标注"() -> (w193:bool)
          n142 = case shown="真" w193 {
            tunnel: [FALSE ("T button?") w199] -> w192
            frame False {
            }
            frame True {
              n143 = Two Button Dialog(message="请确认是否完成标注\n完成标注后只能删除，无法新增标注" ("消息")) -> (T button?=w200:bool)  [unwired: 2 in]
              n144 = case shown="真" w200 {
                selector: w200 -> [_ w204]
                tunnel: [FALSE w204] -> w199
                frame False {
                }
                frame True {
                  w203 = T5."Enabled" ("禁用")
                  n145 = property on="导入图像" class="Bool"("DisabledEnum"=w203) -> ()  [unwired: 2 in, 2 out]
                  n146 = property on="删除标注" class="Bool (严格)"("DisabledEnum"=w203) -> ()  [unwired: 2 in, 2 out]
                  n147 = property on="查看评定结果" class="Bool (严格)"("DisabledEnum"=w203) -> ()  [unwired: 2 in, 2 out]
                  n148 = property on="生成报告" class="Bool"("DisabledEnum"=w203) -> ()  [unwired: 2 in, 2 out]
                }
              }
            }
          }
          n149 = local write "穿透图"(w195) -> ()
          n150 = local write "框组"(w190) -> ()
          n151 = local read "stop"() -> (w194:bool)
          n152 = Or(x=w194, y=w192) -> (x .or. y?=w189:bool)
          n153 = call <vilib>:"Application Directory.vi"() -> ()  [unwired: 1 out]
        }
      }
      event "删除标注": Value Change {
        w272 = T5."Disabled and Grayed Out" ("禁用")
        n154 = event-data() -> ()  [unwired: 1 in, 6 out]
        n155 = call "用户输入2"() -> ("框号"=w273:dbl, "确定"=w274:bool)  [unwired: 17 in, 1 out]
        n156 = property on="生成报告" class="Bool"("DisabledEnum"=T5."Enabled" ("禁用")) -> ()  [unwired: 2 in, 2 out]
        n157 = property on="完成标注" class="Bool (严格)"("DisabledEnum"=w272) -> ()  [unwired: 2 in, 2 out]
        n158 = property on="开始标注" class="Bool"("DisabledEnum"=w272) -> ()  [unwired: 2 in, 2 out]
        n159 = case shown="真" w274 {
          tunnel: w273 -> [_ w275]
          frame False {
            # "用户取消操作"
          }
          frame True {
            n160 = stacked-sequence {
              tunnel: w275 -> [_ w282 _]
              frame #0 {
                # "1. 删除所有框"
                n161 = local read "穿透图"() -> (w276:T1)
                n162 = call "IMAQ Clear Overlay"("Image"=w276) -> ()  [unwired: 9 in, 2 out]
              }
              frame #1 {
                # "2. 删除框组中指定元素"
                n163 = local read "部位信息"() -> (w279:string[])
                n164 = local read "框组"() -> (w281:T3)
                n165 = Decrement(x=w282) -> (x-1=w278:dbl)
                n166 = Delete From Array(array=w279, index=w278) -> (array with subset deleted=w277:string[])  [unwired: 1 in, 1 out]
                n167 = Delete From Array(array=w281, index=w278) -> (array with subset deleted=w280:T3)  [unwired: 1 in, 1 out]
                n168 = local write "框组"(w280) -> ()
                n169 = local write "部位信息"(w277) -> ()
              }
              frame #2 {
                # "3. 重画所有框"
                n170 = while {
                  i -> [w295]
                  stop <- w286 stop-if-true
                  n171 = local read "框组"() -> (w290:T3)
                  n172 = local read "穿透图"() -> (w294:T1)
                  n173 = Array Size(array=w290) -> (size(s)=w291:i32)
                  n174 = Index Array(array=w290, index=w295) -> (element=w285:T6)
                  n175 = Increment(x=w295) -> (x+1=w302:i32)
                  n176 = local write "框数"(w291) -> ()
                  n177 = Greater Or Equal?(x=w302, y=w291) -> (x >= y?=w286:bool)
                  n178 = call "IMAQ Overlay ROI"("ROI Descriptor"=w285, "Image"=w294) -> ("Image Out"=w300:T1)  [unwired: 8 in, 1 out]
                  n179 = Unbundle(w285) -> ("Global Rectangle"=w292:i32[])  [unwired: 1 out]
                  n180 = Number To Decimal String(number=w302) -> (decimal integer string=w287:string)  [unwired: 1 in]
                  n181 = Index Array(array=w292, index=0 ("索引")) -> (element=w297:i32)
                  n182 = Index Array(array=w292, index=1 ("索引")) -> (element=w298:i32)
                  n183 = local read "自定义字体"() -> (w284:T2)
                  n184 = Concatenate Strings(w287, "#" ("字符串")) -> (w283:string)
                  n185 = Bundle(w297, w298) -> (w288:cluster{i32, i32})  [unwired: 1 in]
                  n186 = call "IMAQ Overlay Text"("Text Color (black)"=u32 16711680, "Font, Size & Style"=w284, "String"=w283, "Origin"=w288, "Image"=w300) -> ("Image Out"=w293:T1)  [unwired: 5 in, 1 out]
                  n187 = local write "穿透图"(w293) -> ()
                }
              }
            }
          }
        }
      }
      event "查看评定结果": Value Change {
        w311 = T5."Disabled and Grayed Out" ("禁用")
        # "只读穿透图的图像处理方法"
        # "查看指定框的详细信息，包括灰度和面积阈值分割后的结果，提取到的长宽面积等信息"
        n188 = event-data() -> ()  [unwired: 1 in, 6 out]
        n189 = property on="完成标注" class="Bool (严格)"("DisabledEnum"=w311) -> ()  [unwired: 2 in, 2 out]
        n190 = local read "判定为筋条的长宽比阈值"() -> (w306:i32)
        n191 = property on="开始标注" class="Bool"("DisabledEnum"=w311) -> ()  [unwired: 2 in, 2 out]
        n192 = local read "计入缺陷的面积阈值"() -> (w309:i32)
        n193 = local read "临界面积百分比值"() -> (w313:dbl)
        n194 = local read "计入缺陷的Z值阈值"() -> (w307:i32)
        n195 = local read "图像Y向分辨率（mm/像素）"() -> (w304:dbl)
        n196 = local read "图像X向分辨率（mm/像素）"() -> (w305:dbl)
        n197 = local read "缺陷灰度阈值"() -> (w308:dbl)
        n198 = local read "临界Z值"() -> (w314:i32)
        n199 = local read "部位信息"() -> (w316:string[])
        n200 = local read "穿透图"() -> (w303:T1)
        n201 = local read "框组"() -> (w315:T3)
        n202 = call "子VI-查看某框.vi"("输入框号（默认值0为整张图）"=0.0 ("框号"), "框组"=w315, "判定为筋条的长宽比阈值"=w306, "临界Z值"=w314, "缺陷灰度阈值"=w308, "临界面积百分比值"=w313, "计入缺陷的面积阈值"=w309, "计入缺陷的Z值阈值"=w307, 8:w303, "部位信息"=w316, "图像Y向分辨率（mm/像素）"=w304, "图像X向分辨率（mm/像素）"=w305) -> ("全部检测结果"=→"全部检测结果":string[][])  [unwired: 15 in]
      }
      event "生成报告": Value Change {
        w328 = T5."Disabled and Grayed Out" ("禁用")
        # "相当于“查看标注”一栏中的操作做循环，遍历所有框，\n将输出结果叠加为数组，作为最终结果输出并导入word"
        n203 = event-data() -> ()  [unwired: 1 in, 6 out]
        n204 = call "报告模式选择"() -> ("深度学习方法"=w327:bool, "自动检测结果"=w330:bool, "手动框选结果"=w331:bool, "确定"=w329:bool)  [unwired: 15 in, 1 out]
        n205 = Initialize Array(i8 0 ("元素"), 0 ("维数大小")) -> (w317:i8[])
        n206 = local read "计入缺陷的面积阈值"() -> (w324:i32)
        n207 = Build Array(w331, w330, w327) -> (w333:bool[])
        n208 = local read "判定为筋条的长宽比阈值"() -> (w323:i32)
        n209 = local read "缺陷灰度阈值"() -> (w334:dbl)
        n210 = local read "图像Y向分辨率（mm/像素）"() -> (w321:dbl)
        n211 = local read "临界面积百分比值"() -> (w335:dbl)
        n212 = local read "计入缺陷的Z值阈值"() -> (w325:i32)
        n213 = Boolean Array To Number(Boolean array=w333) -> (number=w332:u32)
        n214 = local read "图像X向分辨率（mm/像素）"() -> (w322:dbl)
        n215 = local read "部位信息"() -> (w338:string[])
        n216 = local read "框组"() -> (w337:T3)
        n217 = property on="删除标注" class="Bool (严格)"("DisabledEnum"=w328) -> ()  [unwired: 2 in, 2 out]
        n218 = property on="完成标注" class="Bool (严格)"("DisabledEnum"=w328) -> ()  [unwired: 2 in, 2 out]
        n219 = property on="开始标注" class="Bool"("DisabledEnum"=w328) -> ()  [unwired: 2 in, 2 out]
        n220 = local read "临界Z值"() -> (w336:i32)
        n221 = local read "穿透图"() -> (w320:T1)
        n222 = case shown="真" w329 {
          tunnel: w338 -> [_ w357]
          tunnel: w337 -> [_ w356]
          tunnel: w336 -> [_ w355]
          tunnel: w335 -> [_ w354]
          tunnel: string[][] [] ("分层类检测结果合并 2") -> [_ w353]
          tunnel: w334 -> [_ w352]
          tunnel: w332 -> [_ w351]
          tunnel: w325 -> [_ w348]
          tunnel: w324 -> [_ w347]
          tunnel: w323 -> [_ w345]
          tunnel: w322 -> [_ w344]
          tunnel: w321 -> [_ w343]
          tunnel: w320 -> [_ w342]
          tunnel: w317 -> [_ w341]
          frame False {
          }
          frame True {
            n223 = case shown="0, 默认" w351 {
              tunnel: [w373 w409 w449 w458] -> w358
              tunnel: w357 -> [w375 w415 w453 _]
              tunnel: w356 -> [w376 w414 w452 _]
              tunnel: w355 -> [w378 w411 w451 w463]
              tunnel: w354 -> [w379 w412 w450 w460]
              tunnel: w353 -> [w380 w410 w448 w465]
              tunnel: w352 -> [w377 w413 w443 w462]
              tunnel: w348 -> [w371 w408 w444 w459]
              tunnel: w347 -> [w370 w407 w445 w461]
              tunnel: w345 -> [w369 w406 w442 w457]
              tunnel: w344 -> [w368 w405 w441 _]
              tunnel: w343 -> [w367 w404 w440 _]
              tunnel: w342 -> [w366 w403 w439 _]
              tunnel: w341 -> [w365 w402 _ _]
              tunnel: [w364 w401 i32[] [] i32[] []] -> w340
              frame 0, Default {
                # "只读穿透图的图像处理方法"
                # "默认手动框选结果"
                n224 = local read "框数"() -> (w374:dbl)
                n225 = for {
                  N: w374 -> [_]
                  shift-right: [w400] -> w373
                  shift-left: w380 -> [w399]
                  tunnel: w375 -> [w398]
                  tunnel: w376 -> [w397]
                  tunnel: w379 -> [w396]
                  tunnel: w377 -> [w391]
                  tunnel: w378 -> [w395]
                  tunnel: w371 -> [w392]
                  tunnel: w370 -> [w393]
                  tunnel: w369 -> [w390]
                  tunnel: w368 -> [w389]
                  tunnel: w367 -> [w388]
                  tunnel: w366 -> [w387]
                  shift-right: [w384] -> w364
                  shift-left: w365 -> [w385]
                  i -> [w381]
                  n226 = Increment(x=w381) -> (x+1=w382:i32)
                  n227 = call "子VI-查看某框-不显示界面.vi"("框号"=w382, "框组"=w397, "计入缺陷的Z值阈值"=w392, "临界Z值"=w395, "计入缺陷的面积阈值"=w393, "临界面积百分比值"=w396, "图像Y向分辨率（mm/像素）"=w388, "缺陷灰度阈值"=w391, 8:w387, "部位信息"=w398, "判定为筋条的长宽比阈值"=w390, "图像X向分辨率（mm/像素）"=w389) -> ("全部检测结果"=w394:string[][], "flag标记簇"=w386:cluster{"框号":dbl, "数值":i32})  [unwired: 14 in]
                  n228 = Unbundle(w386) -> ("数值"=w383:i32)  [unwired: 1 out]
                  n229 = Build Array (concatenate)(w399, w394) -> (w400:string[][])
                  n230 = Build Array (concatenate)(w385, w383) -> (w384:i32[])
                }
                "报告模式" <- "手动框选"
              }
              frame 1 {
                # "只读穿透图的图像处理方法"
                n231 = local write "报告模式"("手动框选") -> ()
                n232 = local read "框数"() -> (w416:dbl)
                n233 = for {
                  N: w416 -> [_]
                  shift-right: [w437] -> w409
                  shift-left: w410 -> [w436]
                  tunnel: w415 -> [w435]
                  tunnel: w414 -> [w434]
                  tunnel: w413 -> [w428]
                  tunnel: w412 -> [w433]
                  tunnel: w411 -> [w432]
                  tunnel: w408 -> [w429]
                  tunnel: w407 -> [w430]
                  tunnel: w406 -> [w427]
                  tunnel: w405 -> [w426]
                  tunnel: w404 -> [w425]
                  tunnel: w403 -> [w424]
                  shift-right: [w422] -> w401
                  shift-left: w402 -> [w421]
                  i -> [w418]
                  n234 = Increment(x=w418) -> (x+1=w419:i32)
                  n235 = call "子VI-查看某框-不显示界面.vi"("框号"=w419, "框组"=w434, "计入缺陷的Z值阈值"=w429, "临界Z值"=w432, "计入缺陷的面积阈值"=w430, "临界面积百分比值"=w433, "图像Y向分辨率（mm/像素）"=w425, "缺陷灰度阈值"=w428, 8:w424, "部位信息"=w435, "判定为筋条的长宽比阈值"=w427, "图像X向分辨率（mm/像素）"=w426) -> ("全部检测结果"=w431:string[][], "flag标记簇"=w423:cluster{"框号":dbl, "数值":i32})  [unwired: 14 in]
                  n236 = Unbundle(w423) -> ("数值"=w420:i32)  [unwired: 1 out]
                  n237 = Build Array (concatenate)(w436, w431) -> (w437:string[][])
                  n238 = Build Array (concatenate)(w421, w420) -> (w422:i32[])
                }
              }
              frame 2 {
                # "只读穿透图的图像处理方法"
                n239 = local write "报告模式"("自动检测") -> ()
                n240 = call "子VI-查看某框-不显示界面.vi"("框号"=0.0, "框组"=w452, "计入缺陷的Z值阈值"=w444, "临界Z值"=w451, "计入缺陷的面积阈值"=w445, "临界面积百分比值"=w450, "图像Y向分辨率（mm/像素）"=w440, "缺陷灰度阈值"=w443, 8:w439, "部位信息"=w453, "判定为筋条的长宽比阈值"=w442, "图像X向分辨率（mm/像素）"=w441) -> ("全部检测结果"=w446:string[][])  [unwired: 14 in, 1 out]
                n241 = Build Array (concatenate)(w448, w446) -> (w449:string[][])
              }
              frame 4 {
                # "深度学习方法自动检测demo"
                n242 = local read "穿透图原始路径"() -> (w456:path)
                n243 = local write "报告模式"("深度学习自动检测" ("报告模式")) -> ()
                n244 = call "子VI-深度学习自动检测.vi"("临界Z值"=w463, "判定为筋条的长宽比阈值"=w457, "临界面积百分比值"=w460, "缺陷灰度阈值"=w462, "计入缺陷的面积阈值"=w461, "穿透图原始路径"=w456, "计入缺陷的Z值阈值"=w459) -> ("全部检测结果"=w464:string[][])  [unwired: 8 in]
                n245 = Build Array (concatenate)(w464, w465) -> (w458:string[][])
              }
            }
            "flag数组" <- w340
            n246 = flat-sequence {
              tunnel: w358 -> [w469]
              tunnel: [w468] -> w346
              tunnel: [w470] -> w363
              tunnel: w346 -> [w470]
              tunnel: w363 -> [w523]
              tunnel: [w523] -> w362
              tunnel: w362 -> [w529]
              tunnel: [w529] -> w361
              tunnel: [w525] -> w350
              tunnel: [w524] -> w349
              tunnel: [w557] -> w360
              tunnel: [w556] -> w359
              tunnel: w361 -> [w550]
              tunnel: w350 -> [w547]
              tunnel: w349 -> [w546]
              tunnel: w359 -> [w575]
              tunnel: w360 -> [w576]
              frame #0 {
                # "2023.7.21\n增加手动修改评定结果子vi\n手动修改类型点击确认再判定和生成报告"
                n247 = local read "临界面积百分比值"() -> (w467:dbl)
                n248 = call "子VI-修改评定结果.vi"("全部检测结果"=w469, "临界面积百分比值"=w467) -> ("全部检测结果合并输出"=w468:string[][])  [unwired: 9 in]
              }
              frame #1 {
                n249 = while {
                  tunnel: [w482] -> _
                  i -> [w472]
                  stop <- w482 stop-if-true
                  # "2023.8.8\n分析框组，如果没有结果，\n不绘制在报告图上"
                  # "生成绘制了ROI的图像\n可以用于后续的图片导出保存"
                  n250 = local read "框组"() -> (w483:T3)
                  n251 = local read "ROImask"() -> (w476:T1)
                  n252 = local read "flag数组"() -> (w479:i8[])
                  n253 = local read "穿透图"() -> (w473:T1)
                  n254 = Array Size(array=w483) -> (size(s)=w484:i32)
                  n255 = Index Array(array=w483, index=w472) -> (element=w475:T6)
                  n256 = Increment(x=w472) -> (x+1=w471:i32)
                  n257 = Index Array(array=w479, index=w472) -> (element=w478:i8)
                  n258 = Greater Or Equal?(x=w471, y=w484) -> (x >= y?=w482:bool)
                  n259 = Equal?(x=w478, y=i8 1) -> (x = y?=w474:bool)
                  n260 = case shown="真" w474 {
                    tunnel: [w486 w503] -> w481
                    tunnel: [errorcluster {"status"=FALSE, "code"=0, "source"=""} ("error out") w491] -> w480
                    tunnel: w476 -> [w486 w490]
                    tunnel: w475 -> [_ w489]
                    tunnel: w473 -> [_ w488]
                    tunnel: w471 -> [_ w487]
                    frame False {
                    }
                    frame True {
                      w509 = 1 items=["White", "Black", "Inverted", "Black on White", "White on Black"] ("Color")
                      w511 = u16 2 items=["Frame", "Paint", "Invert Frame", "Invert Paint"] ("Draw Mode")
                      w506 = u16 1 items=["Line", "Rectangle", "Oval"] ("Shape to draw")
                      n261 = Unbundle By Name(w489) -> ("Global Rectangle"=w498:i32[])
                      n262 = Index Array(array=w498, index=2 ("索引")) -> (element=w497:i32)
                      n263 = Index Array(array=w498, index=0 ("索引")) -> (element=w494:i32)
                      n264 = Index Array(array=w498, index=3 ("索引")) -> (element=w496:i32)
                      n265 = Index Array(array=w498, index=1 ("索引")) -> (element=w493:i32)
                      n266 = Build Array(w494, w493, w497, w496) -> (w495:i32[])
                      n267 = call "IMAQ Draw"("Draw Mode"=w511, "Shape to draw"=w506, "Coordinates"=w495, "Image Src"=w488) -> ("Image Dst Out"=w510:T1)  [unwired: 6 in, 1 out]
                      n268 = Number To Decimal String(number=w487) -> (decimal integer string=w507:string)  [unwired: 1 in]
                      n269 = local read "自定义字体"() -> (w504:T2)
                      n270 = Concatenate Strings(w507, "#" ("字符串")) -> (w505:string)
                      n271 = Build Array(w494, w493) -> (w492:i32[])
                      n272 = call "IMAQ Draw Text"("String"=w505, "Insertion Point"=w492, "Color"=w509, "Font, Size & Style"=w504, "Image Dst"=w490, "Image Src"=w510) -> ("error out"=w491:errorcluster, "Image Dst Out"=w503:T1)  [unwired: 2 in, 2 out]
                      n273 = local write "ROImask"(w503) -> ()
                    }
                  }
                  "ROImask" <- w481
                  n274 = case shown="错误" w480 {
                    frame No Error {
                    }
                    frame Error {
                      n275 = One Button Dialog(message="失败！无法保存图片到报告" ("消息")) -> ()  [unwired: 1 in, 1 out]
                    }
                  }
                }
              }
              frame #2 {
                n276 = local read "穿透图原始路径"() -> (w522:path)
                n277 = local read "ROImask"() -> (w514:T1)
                n278 = Path To String(path=w522) -> (string=w519:string)
                n279 = String Length(string=w519) -> (length=w520:i32)
                n280 = Subtract(x=w520, y=4) -> (x-y=w521:i32)
                n281 = Replace Substring(3:w521, 4:"_标注后.png" ("字符串"), 5:w519) -> (1:w518:string)  [unwired: 1 in, 1 out]
                n282 = String To Path(string=w518) -> (path=w513:path)
                "标注后的图片路径" <- w513
                n283 = call-poly "IMAQ Write File 2"("Image Quality"=u32 1000, "File Path"=w513, "Image"=w514) -> ()  [unwired: 7 in, 2 out]
              }
              frame #3 {
                # "最终检测结果全部合并 导入word中"
                n284 = call <vilib>:"Application Directory.vi"() -> ("Application Directory"=w528:path)
                n285 = Build Path(base path=w528, name or relative path="report-template.docx") -> (appended path=w526:path)
                n286 = call <vilib>:"Create Report.vi"("window state (normal)"=T8."maximized", "report type"=Report_Type."Word", "template (empty)"=w526) -> ("report out"=w525:refnum<class "NI_report.lvclass">, "error out"=w524:errorcluster)  [unwired: 11 in]
              }
              frame #4 {
                n287 = local read "报告模式"() -> (w548:string)
                n288 = local read "质量等级"() -> (w544:string)
                n289 = Get Date/Time String(date format (0)=enum16{"short", "long", "abbreviated"}."long" ("日期格式(0)")) -> (date string=w554:string, time string=w555:string)  [unwired: 2 in]
                n290 = call-poly <vilib>:"Append Report Text.vi"("report in"=w547, "MS Office parameters"=T12 {"position (excel)"={"row"=0, "column"=0}, "name (excel)"="", "bookmark (word)"="mode"}, "text"=w548, "error in (no error)"=w546) -> ("report out"=w543:refnum<class "NI_report.lvclass">, "error out"=w542:errorcluster)  [unwired: 8 in, 2 out]
                n291 = Concatenate Strings(w554, w555) -> (w553:string)
                n292 = local read "标注后的图片路径"() -> (w537:path)
                n293 = call-poly <vilib>:"Append Report Text.vi"("report in"=w543, "MS Office parameters"=T12 {"position (excel)"={"row"=0, "column"=0}, "name (excel)"="", "bookmark (word)"="class"}, "text"=w544, "error in (no error)"=w542) -> ("report out"=w540:refnum<class "NI_report.lvclass">, "error out"=w541:errorcluster)  [unwired: 8 in, 2 out]
                n294 = call-poly <vilib>:"Append Report Text.vi"("report in"=w540, "MS Office parameters"=T12 {"position (excel)"={"row"=0, "column"=0}, "name (excel)"="", "bookmark (word)"="time"}, "text"=w553, "error in (no error)"=w541) -> ("report out"=w534:refnum<class "NI_report.lvclass">, "error out"=w535:errorcluster)  [unwired: 8 in, 2 out]
                n295 = call-poly <vilib>:"Append Image to Report.vi"("report in"=w534, "alignment (default)"=HTML_Report_Image_Alignment."MIDDLE", "MS Office parameters"=T11 {"position (Excel)"={"row"=0, "column"=0}, "name (Excel)"="", "bookmark (Word)"="image"}, "path or URL of image"=w537) -> ("report out"=w533:refnum<class "NI_report.lvclass">, "error out"=w536:errorcluster)  [unwired: 8 in, 2 out]
                n296 = call <vilib>:"Word Easy Text.vi"("report in"=w533, "text"="检测结果：", "alignment (left)"=enum16{"Left", "Centered", "Right", "Justify"}."Left", "font"=T13 {"font name"="", "font size"=0.0, "bold"=0, "italic"=0, "underline"=0, "strike through"=0, "font color"=16777216}, "error in (no error)"=w535) -> ("report out"=w532:refnum<class "NI_report.lvclass">, "error out"=w559:errorcluster)  [unwired: 8 in, 1 out]
                n297 = call-poly <vilib>:"Word Easy Table.vi"("report in"=w532, "column headers"=string[] ["框号", "X/mm", "Y/mm", "长/mm", "宽/mm", "面积/mm2", "Z值/mm", "部位", "类型", "合格性", "缺陷序号"], "data"=w550, "error in (no error)"=w559) -> ("report out"=w557:refnum<class "NI_report.lvclass">, "error out"=w556:errorcluster)  [unwired: 9 in, 1 out]
                n298 = case shown="错误" w536 {
                  frame No Error {
                  }
                  frame Error {
                    n299 = One Button Dialog(message="图片导入word\n发生错误！" ("消息")) -> ()  [unwired: 1 in, 1 out]
                  }
                }
              }
              frame #5 {
                n300 = local read "穿透图原始路径"() -> (w568:path)
                n301 = local read "报告模式"() -> (w566:string)
                n302 = Path To String(path=w568) -> (string=w572:string)
                n303 = String Length(string=w572) -> (length=w573:i32)
                n304 = Subtract(x=w573, y=4) -> (x-y=w574:i32)
                n305 = Concatenate Strings("_" ("字符串"), w566, ".docx" ("字符串")) -> (w564:string)
                n306 = Replace Substring(3:w574, 4:w564, 5:w572) -> (1:w571:string)  [unwired: 1 in, 1 out]
                n307 = String To Path(string=w571) -> (path=w569:path)
                "添加的路径" <- w569
                n308 = call-dynamic "Save Report to File.vi"("report in"=w576, "report file path"=w569, "prompt to replace? (F)"=TRUE, "error in (no error)"=w575) -> ("report out"=w580:refnum<class "NI_report.lvclass">, "error out"=w579:errorcluster)  [unwired: 10 in]
                n309 = call <vilib>:"Word Bring to Front.vi"("report in"=w580, "window state (maximized)"=enum16{"maximized", "minimized", "normal"}."normal", "error in (no error)"=w579) -> ()  [unwired: 11 in, 2 out]
              }
              frame #6 {
                n310 = local write "全部检测结果合并"(string[][] [] ("弥散类检测结果合并")) -> ()
                n311 = One Button Dialog(message="完成评定并退出程序！\n请查看word报告" ("消息")) -> ()  [unwired: 1 in, 1 out]
              }
            }
          }
        }
      }
      event "stop": Value Change {
        # "退出软件"
        n312 = event-data() -> ("NewVal"=w586:bool)  [unwired: 1 in, 4 out]
        n313 = Two Button Dialog(message="是否关闭本软件？" ("消息")) -> (T button?=w587:bool)  [unwired: 2 in]
        n314 = And(x=w586, y=w587) -> (x .and. y?=w585:bool)
        n315 = case shown="真" w585 {
          frame False {
          }
          frame True {
            n316 = local read "穿透图"() -> (w589:T1)
            n317 = call "Imaq Dispose"("All Images? (No)"=TRUE, "Image"=w589) -> ()  [unwired: 4 in, 1 out]
            n318 = disable-structure shown="RUN_TIME_ENGINE==True" {
              frame condition #0 {
                n319 = Quit LabVIEW() -> ()  [unwired: 1 in]
              }
              frame condition #1 (active) {
                n320 = Stop() -> ()  [unwired: 1 in]
              }
            }
          }
        }
      }
    }
  }
  n321 = disable-structure shown="启用" {
    frame Disabled {
      n322 = while {
        stop <- FALSE stop-if-true
        n323 = local read "查看评定结果"() -> (w592:bool)
        n324 = local read "删除标注"() -> (w593:bool)
        n325 = Or(x=w593, y=w592) -> (x .or. y?=w594:bool)
        n326 = local write "开始标注"(w594) -> ()
        n327 = Wait Until Next ms Multiple(millisecond multiple=u32 50 ("毫秒倍数")) -> ()  [unwired: 1 out]
      }
    }
    frame Enabled {
    }
  }
  n328 = disable-structure shown="启用" {
    frame Disabled {
    }
    frame Enabled {
    }
  }
  "临界面积百分比值" <- w15
  "缺陷灰度阈值" <- w16
